vi "SystemLink Server selector.vi"() -> ()   [LabVIEW 2017]
uses:
  support/sl_server_selector_states.ctl
  <vilib>/Skyline/Utilities/NI Skyline Utilities.lvlib
panel:
  in  "Refresh":bool
  out "error":errorcluster
  in  "Apply":bool
  out "Hostname (System Name)":string
  out "Current SystemLink Server for Local System":string
  in  "New SystemLink Server":string(combo)
  # "Current Settings for Local System"
  # "Change SystemLink Server for Local System"
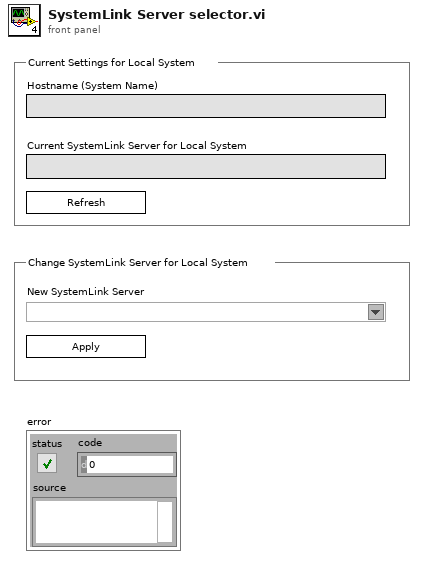
[diagram p1: front panel]
types:
  T1 = typedef "sl_server_selector_states.ctl" = enum16{"Initialize", "Wait for Event", "Exit"}
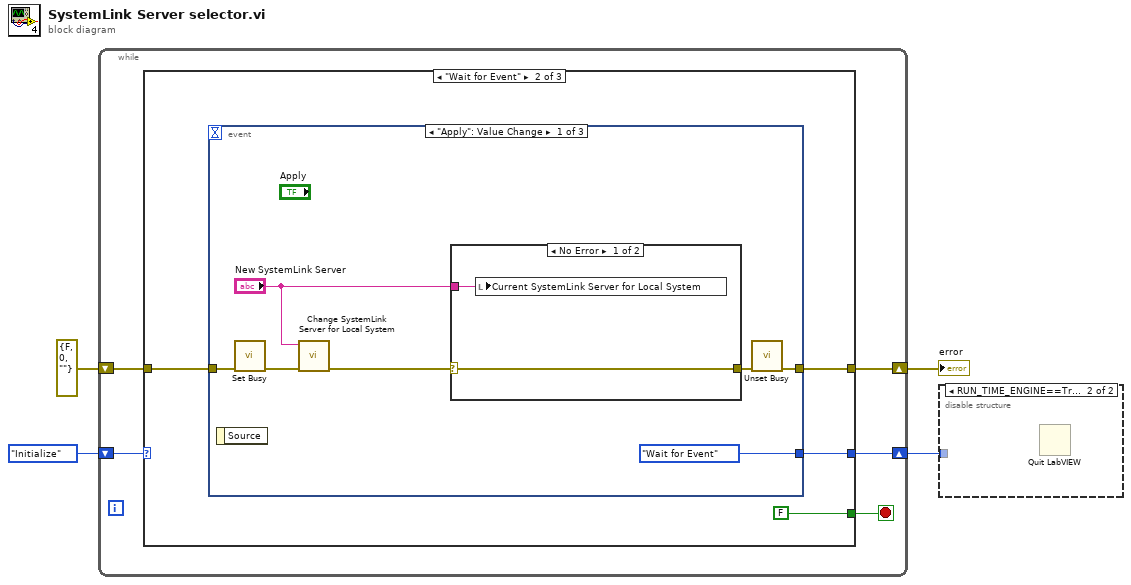
[diagram p0: block diagram]
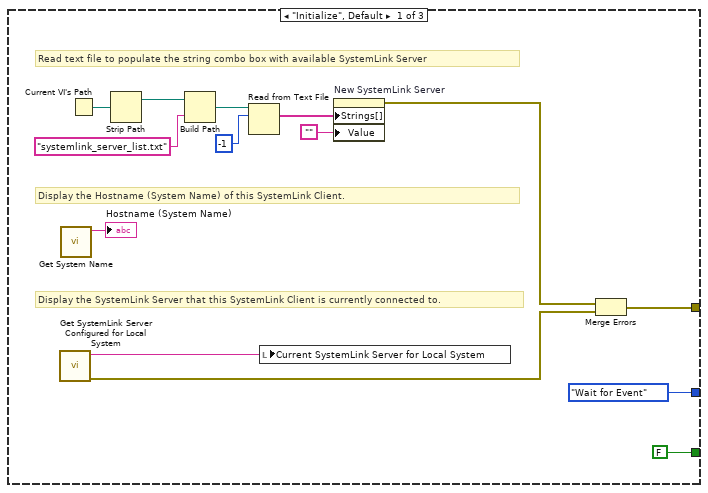
[diagram p2: hidden frame]
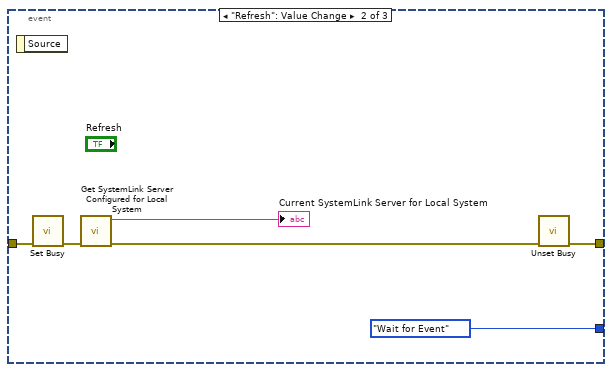
[diagram p4: hidden frame]
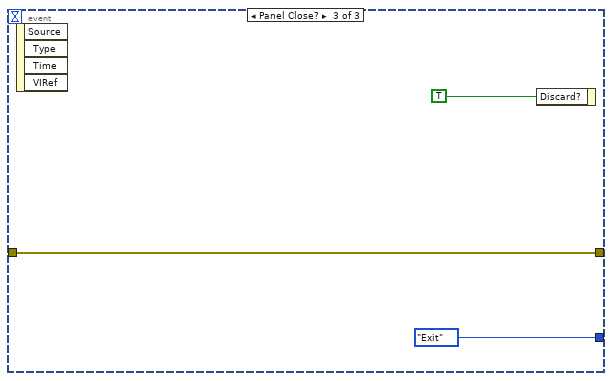
[diagram p5: hidden frame]
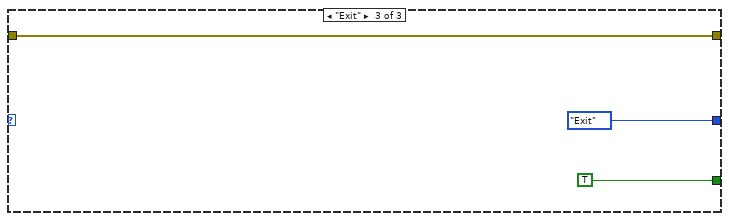
[diagram p6: hidden frame]
diagram:
  n1 = while {
    shift-right: [w8] -> w3
    shift-left: sl_server_selector_states."Initialize" -> [w9]
    shift-right: [w5] -> w1
    shift-left: errorcluster {"status"=FALSE, "code"=0, "source"=""} ("error constant") -> [w6]
    stop <- w7 stop-if-true
    n2 = case shown="\"Wait for Event\"" w9 {
      tunnel: [sl_server_selector_states."Wait for Event" w27 sl_server_selector_states."Exit"] -> w8
      tunnel: [FALSE FALSE TRUE] -> w7
      tunnel: w6 -> [_ w25 w47]
      tunnel: [w17 w24 w47] -> w5
      frame "Initialize", Default {
        # "Read text file to populate the string combo box with available SystemLink Server"
        # "Display the Hostname (System Name) of this SystemLink Client."
        # "Display the SystemLink Server that this SystemLink Client is currently connected to."
        n3 = call "Get SystemLink Server Configured for Local System.vi"() -> ("error out"=w13:errorcluster, "SystemLink Server Configured for Local System"=w12:string)  [unwired: 10 in]
        n4 = call <vilib>:"Get System Name.vi"() -> ("system name"=→"Hostname (System Name)":string)  [unwired: 11 in]
        n5 = Current VI's Path() -> (path=w22:path)
        n6 = Strip Path(path=w22) -> (stripped path=w23:path)  [unwired: 1 out]
        n7 = Build Path(base path=w23, name or relative path="systemlink_server_list.txt") -> (appended path=w16:path)
        n8 = Read from Text File(file (use dialog)=w16, count=-1) -> (text=w14:string[])  [unwired: 2 in, 3 out]
        n9 = local write "Current SystemLink Server for Local System"(w12) -> ()
        n10 = property on="New SystemLink Server" class="CmbBox"("Strings[]"=w14, "Value"="") -> (error out=w18:errorcluster)  [unwired: 2 in, 1 out]
        n11 = Merge Errors(w18, w13) -> (w17:errorcluster)
      }
      frame "Wait for Event" {
        n12 = event shown="[0] \"Apply\": Value Change" {
          selector: _ -> [_ _ _]
          dyn-events: _ -> [_ _ _]
          timeout: _ -> [_ _ _]
          tunnel: [sl_server_selector_states."Wait for Event" sl_server_selector_states."Wait for Event" sl_server_selector_states."Exit"] -> w27
          tunnel: w25 -> [w33 w42 w44]
          tunnel: [w31 w38 w44] -> w24
          event "Apply": Value Change {
            n13 = event-data() -> ()  [unwired: 1 in, 1 out]
            n14 = call <vilib>:"Set Busy.vi"("error in (no error)"=w33) -> ("error out"=w32:errorcluster)  [unwired: 9 in, 1 out]
            n15 = call "Change SystemLink Server for Local System.vi"("error in (no error)"=w32, "New SystemLink Server"="New SystemLink Server") -> ("error out"=w30:errorcluster)  [unwired: 9 in]
            n16 = case shown="No Error" w30 {
              selector: w30 -> [w36 w37]
              tunnel: [w36 w37] -> w29
              tunnel: "New SystemLink Server" -> [w35 _]
              frame No Error {
                n17 = local write "Current SystemLink Server for Local System"(w35) -> ()
              }
              frame Error {
              }
            }
            n18 = call <vilib>:"Unset Busy.vi"("error in (no error)"=w29) -> ("error out"=w31:errorcluster)  [unwired: 10 in]
          }
          event "Refresh": Value Change {
            n19 = event-data() -> ()  [unwired: 1 in, 1 out]
            n20 = call <vilib>:"Set Busy.vi"("error in (no error)"=w42) -> ("error out"=w39:errorcluster)  [unwired: 9 in, 1 out]
            n21 = call "Get SystemLink Server Configured for Local System.vi"("error in (no error)"=w39) -> ("error out"=w41:errorcluster, "SystemLink Server Configured for Local System"=→"Current SystemLink Server for Local System":string)  [unwired: 9 in]
            n22 = call <vilib>:"Unset Busy.vi"("error in (no error)"=w41) -> ("error out"=w38:errorcluster)  [unwired: 10 in]
          }
          event Panel Close? {
            n23 = event-data() -> ()  [unwired: 1 in, 4 out]
            n24 = event-data("Discard?"=TRUE) -> ()  [unwired: 1 in, 1 out]
          }
        }
      }
      frame "Exit" {
      }
    }
  }
  "error" <- w1
  n25 = disable-structure shown="RUN_TIME_ENGINE==True" {
    disable-tunnel: w3 -> [_ _]
    frame condition #0 (active) {
    }
    frame condition #1 {
      n26 = Quit LabVIEW() -> ()  [unwired: 1 in]
    }
  }
